vi "Several_loops_prod-cons_23.vi"() -> ()   [LabVIEW 2022 SP3]
doc: "Demo VI, it implements producer-consumer principle for building asynchronous program"
uses:
  27b86aa0-25c0-40d3-a974-310fc08e437a.vi
  4652784b-b2c9-4b62-9975-14206a9570d8.vi
panel:
  out "Loop # 2":string
  out "Loop # 1":string
  in  "Stop":bool
  in  "Action":bool
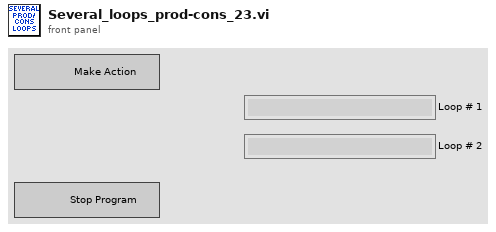
[diagram p1: front panel]
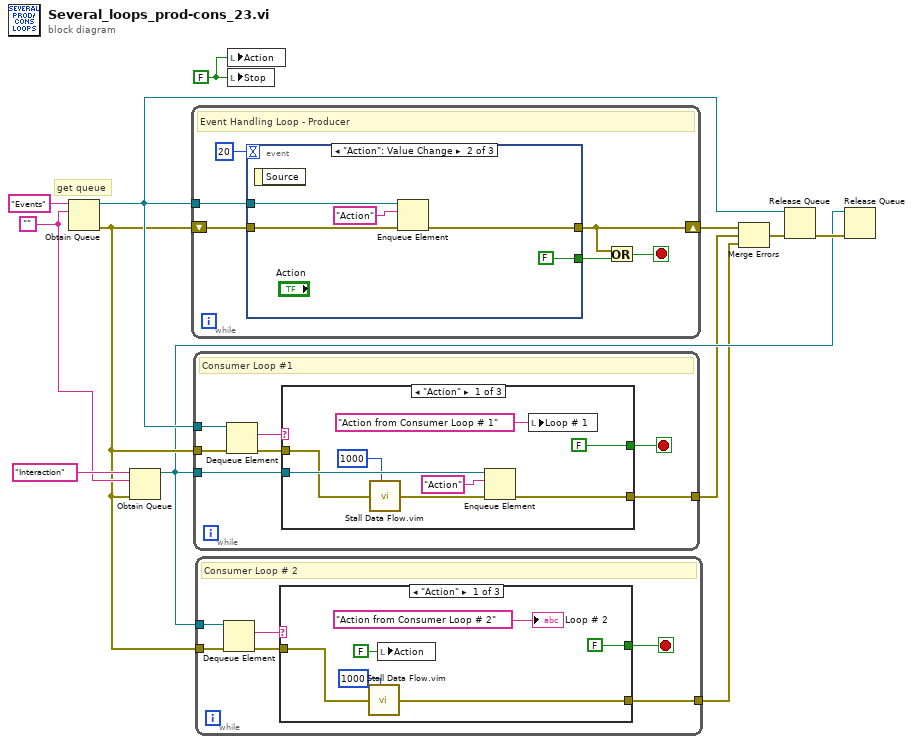
[diagram p0: block diagram]
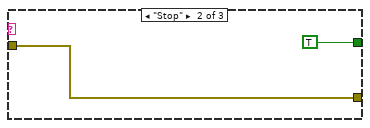
[diagram p2: hidden frame]
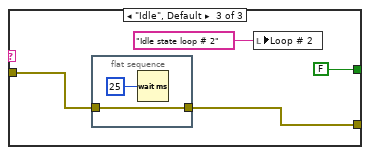
[diagram p3: hidden frame]
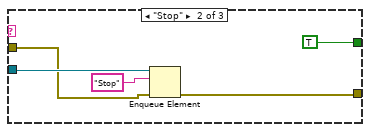
[diagram p4: hidden frame]
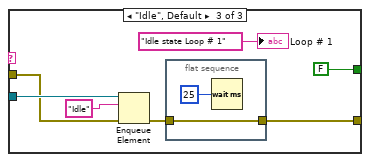
[diagram p5: hidden frame]
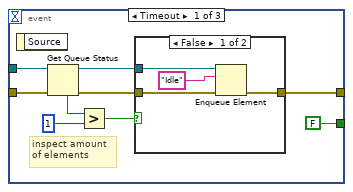
[diagram p6: hidden frame]
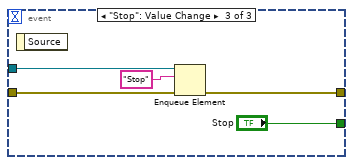
[diagram p8: hidden frame]
diagram:
  w8 = ""
  w12 = FALSE ("Stop")
  # "get queue"
  n1 = Obtain Queue(name (unnamed)="Events", element data type=w8) -> (queue out=w10:refnum<queue>, error out=w6:errorcluster)  [unwired: 3 in, 1 out]
  n2 = Obtain Queue(name (unnamed)="Interaction", element data type=w8, error in (no error)=w6) -> (queue out=w5:refnum<queue>)  [unwired: 2 in, 2 out]
  n3 = while {
    tunnel: w10 -> [w17]
    shift-right: [w15] -> w4
    shift-left: w6 -> [w16]
    stop <- w13 stop-if-true
    # "Event Handling Loop - Producer"
    n4 = event shown="[1] \"Action\": Value Change" {
      selector: _ -> [_ _ _]
      dyn-events: _ -> [_ _ _]
      timeout: 20 -> [_ _ _]
      tunnel: w17 -> [w27 w36 w40]
      tunnel: w16 -> [w26 w37 w41]
      tunnel: [w20 w34 w38] -> w15
      tunnel: [FALSE FALSE ("Stop") "Stop"] -> w14
      event Timeout {
        # "inspect amount\nof elements"
        n5 = event-data() -> ()  [unwired: 1 in, 1 out]
        n6 = Get Queue Status(queue=w27, error in (no error)=w26) -> (queue out=w23:refnum<queue>, error out=w22:errorcluster, # elements in queue=w25:i32)  [unwired: 1 in, 5 out]
        n7 = Greater?(x=w25, y=1) -> (0:w21:bool)
        n8 = case shown="False" w21 {
          tunnel: w23 -> [w31 _]
          tunnel: w22 -> [w29 w32]
          tunnel: [w28 w32] -> w20
          frame False {
            n9 = Enqueue Element(queue=w31, element="Idle", error in (no error)=w29) -> (error out=w28:errorcluster)  [unwired: 1 in, 2 out]
          }
          frame True {
          }
        }
      }
      event "Action": Value Change {
        n10 = event-data() -> ()  [unwired: 1 in, 1 out]
        n11 = Enqueue Element(queue=w36, element="Action", error in (no error)=w37) -> (error out=w34:errorcluster)  [unwired: 1 in, 2 out]
      }
      event "Stop": Value Change {
        n12 = event-data() -> ()  [unwired: 1 in, 1 out]
        n13 = Enqueue Element(queue=w40, element="Stop", error in (no error)=w41) -> (error out=w38:errorcluster)  [unwired: 1 in, 2 out]
      }
    }
    n14 = Or(x=w15, y=w14) -> (x .or. y?=w13:bool)
  }
  n15 = while {
    tunnel: w10 -> [w49]
    tunnel: w6 -> [w48]
    tunnel: w5 -> [w44]
    tunnel: [w43] -> w3
    stop <- w45 stop-if-true
    # "Consumer Loop #1"
    n16 = Dequeue Element(queue=w49, error in (no error)=w48) -> (element=w47:string, error out=w46:errorcluster)  [unwired: 1 in, 2 out]
    n17 = case shown="\"Action\"" w47 {
      tunnel: w46 -> [w53 w59 w66]
      tunnel: [FALSE TRUE FALSE] -> w45
      tunnel: w44 -> [w55 w61 w67]
      tunnel: [w50 w58 w63] -> w43
      frame "Action" {
        n18 = call "Stall Data Flow.vim"("value in"=w53, "milliseconds to wait"=u32 1000) -> ("value out"=w52:errorcluster)  [unwired: 1 out]
        n19 = Enqueue Element(queue=w55, element="Action", error in (no error)=w52) -> (error out=w50:errorcluster)  [unwired: 1 in, 2 out]
        n20 = local write "Loop # 1"("Action from Consumer Loop # 1" ("Answer")) -> ()
      }
      frame "Stop" {
        n21 = Enqueue Element(queue=w61, element="Stop", error in (no error)=w59) -> (error out=w58:errorcluster)  [unwired: 1 in, 2 out]
      }
      frame "Idle", Default {
        n22 = Enqueue Element(queue=w67, element="Idle", error in (no error)=w66) -> (error out=w64:errorcluster)  [unwired: 1 in, 2 out]
        n23 = flat-sequence {
          tunnel: w64 -> [w70]
          tunnel: [w70] -> w63
          frame #0 {
            n24 = Wait (ms)(milliseconds to wait=u32 25) -> ()  [unwired: 1 out]
          }
        }
        "Loop # 1" <- "Idle state Loop # 1" ("Answer")
      }
    }
  }
  n25 = while {
    tunnel: w6 -> [w77]
    tunnel: w5 -> [w76]
    tunnel: [w72] -> w1
    stop <- w73 stop-if-true
    # "Consumer Loop # 2"
    n26 = Dequeue Element(queue=w76, error in (no error)=w77) -> (element=w74:string, error out=w75:errorcluster)  [unwired: 1 in, 2 out]
    n27 = case shown="\"Action\"" w74 {
      tunnel: [FALSE TRUE FALSE] -> w73
      tunnel: w75 -> [w81 w84 w88]
      tunnel: [w80 w84 w87] -> w72
      frame "Action" {
        n28 = call "Stall Data Flow.vim"("value in"=w81, "milliseconds to wait"=u32 1000) -> ("value out"=w80:errorcluster)  [unwired: 1 out]
        n29 = local write "Action"(FALSE ("Action")) -> ()
        "Loop # 2" <- "Action from Consumer Loop # 2" ("Answer")
      }
      frame "Stop" {
      }
      frame "Idle", Default {
        n30 = flat-sequence {
          tunnel: w88 -> [w90]
          tunnel: [w90] -> w87
          frame #0 {
            n31 = Wait (ms)(milliseconds to wait=u32 25) -> ()  [unwired: 1 out]
          }
        }
        n32 = local write "Loop # 2"("Idle state loop # 2" ("Loop # 2")) -> ()
      }
    }
  }
  n33 = local write "Action"(w12) -> ()
  n34 = local write "Stop"(w12) -> ()
  n35 = Merge Errors(w4, w3, w1) -> (w2:errorcluster)
  n36 = Release Queue(queue=w10, error in (no error)=w2) -> (error out=w7:errorcluster)  [unwired: 1 in, 2 out]
  n37 = Release Queue(queue=w5, error in (no error)=w7) -> ()  [unwired: 1 in, 3 out]
